vi "Close All.vi"(8 "error in (no error)":errorcluster, 9 "Interlock Chain":refnum<class "Interlock Chain.lvclass">, 11 "Sample Line in":refnum<class "Sample Line.lvclass">) -> (0 "error out":errorcluster, 3 "Sample Line out":refnum<class "Sample Line.lvclass">)   [LabVIEW 2015, in "cRIO-Carbondioxide.lvlib" / "CO2-Actor.lvlib" / "Sample Line.lvclass"]
uses:
  Sample Line.lvclass
  Interlocks/Interlock Chain/Interlock Chain.lvclass
  <vilib>/ActorFramework/Actor/Actor.lvclass/Actor.ctl
  <vilib>/ActorFramework/Message Enqueuer/Message Enqueuer.lvclass/Message Enqueuer.ctl
  Controls/Sample Line State Enumerator.ctl
  Sample Line.lvclass/Sample Line.ctl
  Valve Messages/Write Bit Field Msg/Write Bit Field Msg.lvclass/Write Bit Field Msg.ctl
  CO2 Actor Messages/Wait Msg/Wait Msg.lvclass/Wait Msg.ctl
  Sample Line Messages/Set Line Status Msg/Set Line Status Msg.lvclass/Set Line Status Msg.ctl
  <vilib>/ActorFramework/Actor/Read Self Enqueuer.vi
  <vilib>/ActorFramework/Message Enqueuer/Enqueue.vi
  <vilib>/ActorFramework/Message Enqueuer/Init from Existing Queue.vi
  <vilib>/ActorFramework/Message Priority Queue/Priority Enqueue.vi
  <vilib>/ActorFramework/Actor/Actor.lvclass
  <vilib>/ActorFramework/Message Enqueuer/Message Enqueuer.lvclass
  Valve Messages/Write Bit Field Msg/Write Bit Field Msg.lvclass
  CO2 Actor Messages/Wait Msg/Wait Msg.lvclass
  Sample Line Messages/Set Line Status Msg/Set Line Status Msg.lvclass
  CO2 Actor/CO2 Actor.lvclass
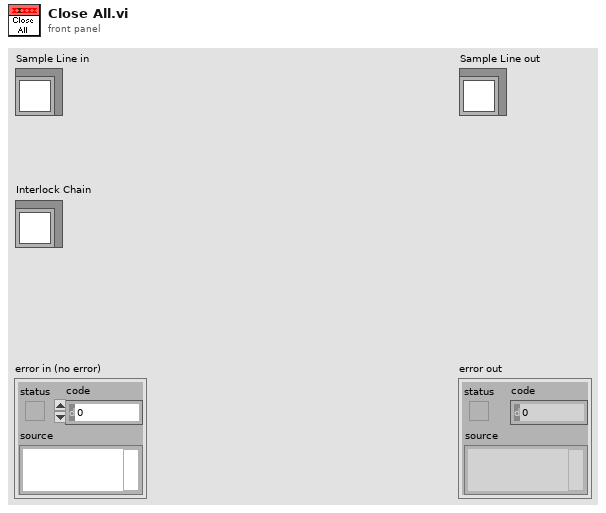
[diagram p1: front panel]
types:
  T1 = typedef "Sample Line State Enumerator.ctl" = enum16{"All lines closed", "Sample line 1.", "Sample line 2.", "Sample line 3.", "Sample line 4.", "Sample line 5.", "Out of range"}
  T2 = cluster{"Valve 1":refnum<class "Message Enqueuer.lvclass">, "Valve 2":refnum<class "Message Enqueuer.lvclass">, "Valve 3":refnum<class "Message Enqueuer.lvclass">, "Valve 4":refnum<class "Message Enqueuer.lvclass">, "Valve 5":refnum<class "Message Enqueuer.lvclass">}
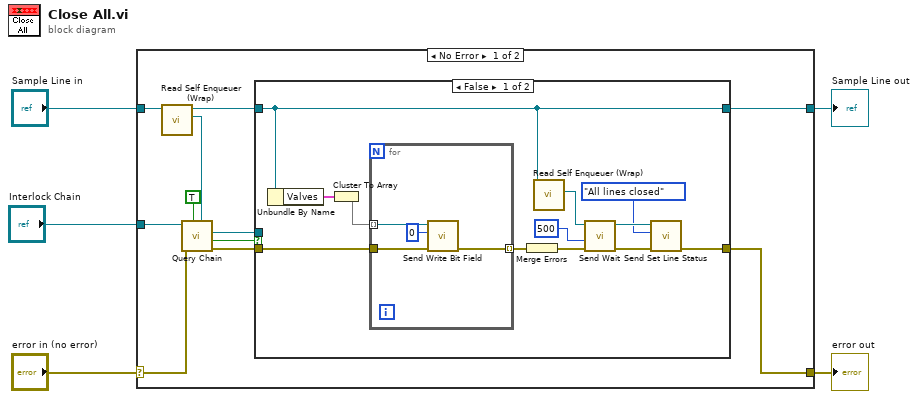
[diagram p0: block diagram]
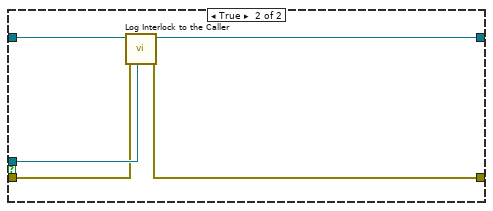
[diagram p2: hidden frame]
diagram:
  n1 = case shown="No Error" "error in (no error)" {
    selector: "error in (no error)" -> [w13 w39]
    tunnel: [w16 w39] -> w4
    tunnel: [w9 w38] -> w2
    tunnel: "Sample Line in" -> [w8 w38]
    tunnel: "Interlock Chain" -> [w15 _]
    frame No Error {
      n2 = call "Read Self Enqueuer (Wrap).vi"("CO2 Actor in"=w8) -> ("Actor Framework:Message Enqueuer"=w6:refnum<class "Message Enqueuer.lvclass">, "CO2 Actor out"=w7:refnum<class "Sample Line.lvclass">)  [unwired: 9 in]
      n3 = call "Query Chain.vi"("Caller Enqueuer"=w6, "Close Connections (F)"=TRUE ("Close Connections if No Interlock (F)"), "error in (no error)"=w13, "Interlock Chain"=w15) -> ("error out"=w12:errorcluster, "Interlock?"=w11:bool, "Interlock out"=w10:refnum<class "Interlock.lvclass">)  [unwired: 2 in, 3 out]
      n4 = case shown="False" w11 {
        tunnel: w7 -> [w19 w36]
        tunnel: [w21 w33] -> w16
        tunnel: w12 -> [w25 w34]
        tunnel: w10 -> [_ w37]
        tunnel: [w19 w35] -> w9
        frame False {
          n5 = Unbundle By Name(w19) -> ("Valves"=w28:T2)
          n6 = Cluster To Array(cluster=w28) -> (array=w27:refnum<class "Message Enqueuer.lvclass">[])
          n7 = for {
            tunnel: w27 -> [w32] mode=indexing
            tunnel: w25 -> [w31]
            tunnel: [w30] -> w26 mode=indexing
            n8 = call "Send Write Bit Field.vi"("error in (no error)"=w31, "Bit Field"=u16 0, "Message Enqueuer"=w32) -> ("error out"=w30:errorcluster)  [unwired: 5 in, 3 out]
          }
          n9 = Merge Errors(w26) -> (w22:errorcluster)
          n10 = call "Read Self Enqueuer (Wrap).vi"("CO2 Actor in"=w19) -> ("Actor Framework:Message Enqueuer"=w17:refnum<class "Message Enqueuer.lvclass">)  [unwired: 9 in, 1 out]
          n11 = call "Send Wait.vi"("error in (no error)"=w22, "milliseconds to wait"=u32 500, "Message Enqueuer"=w17) -> ("error out"=w20:errorcluster, "Message Enqueuer out"=w24:refnum<class "Message Enqueuer.lvclass">)  [unwired: 7 in]
          n12 = call "Send Set Line Status.vi"("error in (no error)"=w20, "Status (All Closed)"=Sample_Line_State_Enumerator."All lines closed", "Message Enqueuer"=w24) -> ("error out"=w21:errorcluster)  [unwired: 7 in, 1 out]
        }
        frame True {
          n13 = call-dynamic "Log Interlock to the Caller.vi"("Interlock in"=w37, "error in (no error)"=w34, "CO2 Actor in"=w36) -> ("error out"=w33:errorcluster, "CO2 Actor out"=w35:refnum<class "Sample Line.lvclass">)  [unwired: 7 in]
        }
      }
    }
    frame Error {
    }
  }
  "error out" <- w4
  "Sample Line out" <- w2
